vi "setRun.vi"() -> ()   [LabVIEW 2017]
panel:
  out "number 2":u32(colorbox)
  in  "String":string
  out "number":u32(colorbox)
  out "hex integer string":string
  in  "Color Box":u32(colorbox)
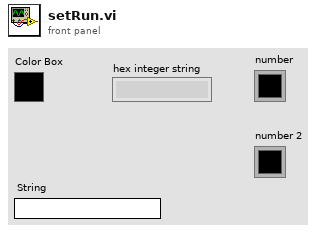
[diagram p1: front panel]
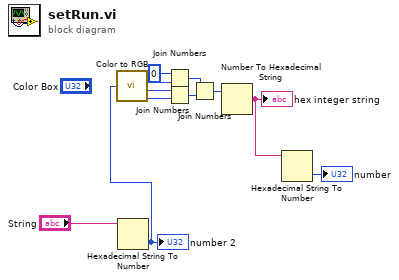
[diagram p0: block diagram]
diagram:
  n1 = Hexadecimal String To Number(string="String") -> (number=w1:u32)  [unwired: 2 in, 1 out]
  "number 2" <- w1
  n2 = call <vilib>:"Color to RGB.vi"("Color"=w1) -> ("R"=w11:u8, "G"=w10:u8, "B"=w9:u8)  [unwired: 1 out]
  n3 = Join Numbers(hi=u8 0, lo=w11) -> ((hi.lo)=w7:u16)
  n4 = Join Numbers(hi=w10, lo=w9) -> ((hi.lo)=w6:u16)
  n5 = Join Numbers(hi=w7, lo=w6) -> ((hi.lo)=w5:u32)
  n6 = Number To Hexadecimal String(2:w5) -> (0:w4:string)  [unwired: 1 in]
  "hex integer string" <- w4
  n7 = Hexadecimal String To Number(string=w4) -> (number=→"number":u32)  [unwired: 2 in, 1 out]
